vi "processData.vi"(8 "error in (no error)":errorcluster, 10 "model":refnum<class "Model.lvclass">, 11 "TestingState in":refnum<class "TestingState.lvclass">) -> (0 "error out":errorcluster, 2 "model 2":refnum<class "Model.lvclass">, 3 "TestingState out":refnum<class "TestingState.lvclass">)   [LabVIEW 2015, in "TestingState.lvclass"]
uses:
  TestingState.lvclass
  Model/Model/Model.lvclass
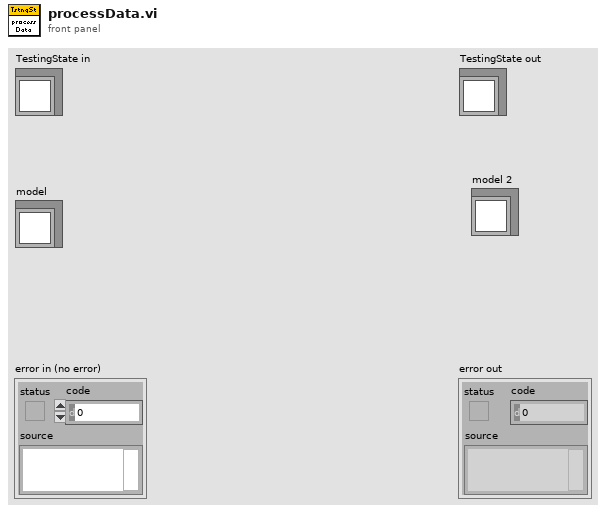
[diagram p1: front panel]
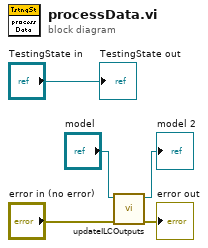
[diagram p0: block diagram]
diagram:
  n1 = call "updateILCOutputs.vi"("error in (no error)"="error in (no error)", "Model in"="model") -> ("error out"=→"error out":errorcluster, "Model out"=→"model 2":refnum<class "Model.lvclass">)  [unwired: 8 in]
  "TestingState out" <- "TestingState in"
